vi "Keithley 2600 Series Read Resistance Measurement.vi"() -> ()   [LabVIEW 2020]
doc: "This example shows how to configure the source output, source measurement and perform one resistance measurement."
uses:
  <instrlib>/Keithley 2600 Series/Public/Configure/Source/Configure Source (Range).vi
  <instrlib>/Keithley 2600 Series/Public/Configure/Source/Configure Source (Level).vi
  <instrlib>/Keithley 2600 Series/Public/Configure/Source/Configure Source (Limit).vi
  <instrlib>/Keithley 2600 Series/Public/Data/Read Measurement (Resistance).vi
  <instrlib>/Keithley 2600 Series/Keithley 2600 Series.lvlib
panel:
  out "Resistance (Ohm)":dbl
  in  "Sense Mode (0: Local Sense)":i32(ring) items=["Local Sense", "Remote Sense"]
  in  "Voltage Limit (5 V)":dbl=5.0
  in  "Current Level (0.1 A)":dbl=0.1
  in  "Current Range (0.1 A)":dbl=0.1
  in  "Source Function (0: Current)":i32(ring) items=["Current"]
  in  "Source Measure Unit Channel (0: Channel A)":i32(ring) items=["Channel A", "Channel B"]
  in  "VISA resource name":refnum<visa-resource-name>
  # "(c) 2020 National Instruments.  ALL RIGHTS RESERVED."
  # "Measurement Result"
  # "Source Output Configuration"
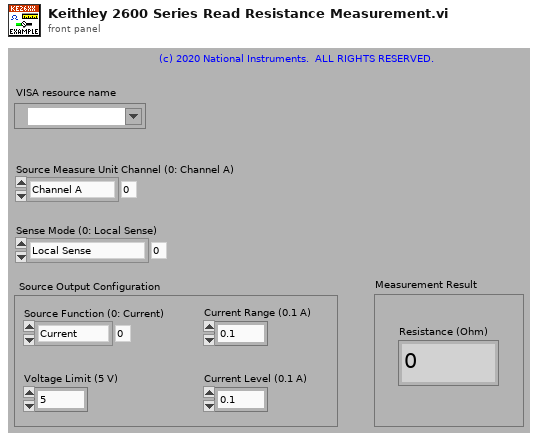
[diagram p1: front panel]
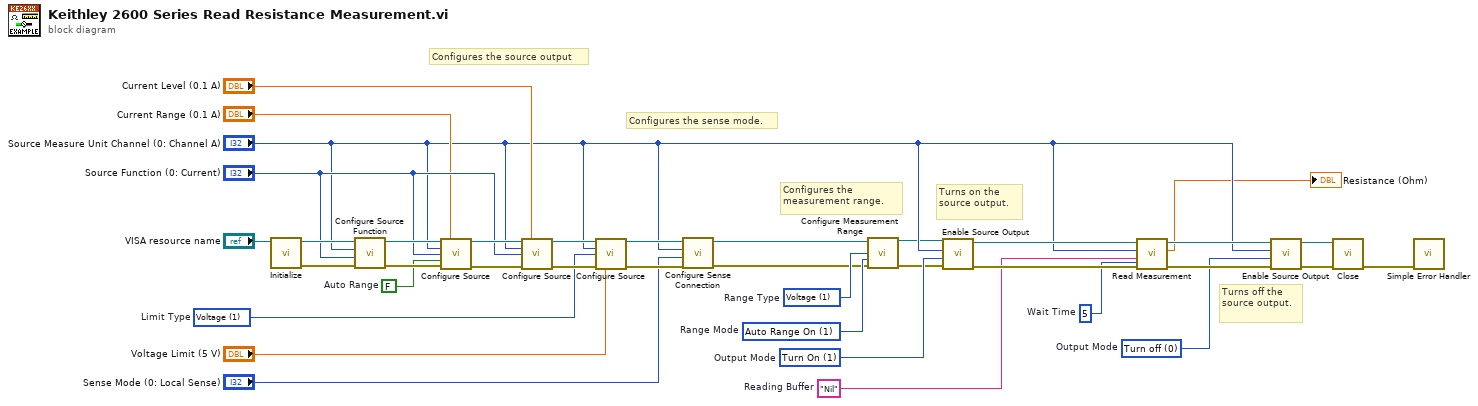
[diagram p0: block diagram]
diagram:
  w1 = 1 items=["Current", "Voltage", "Power"]  # Limit Type
  w9 = 1 items=["Auto Range Off", "Auto Range On", "Auto Range Follow Limit"]  # Range Mode
  w10 = 1 items=["Current", "Voltage"]  # Range Type
  w19 = 0 items=["Turn off", "Turn On", "High-Z"]  # Output Mode
  w22 = 5  # Wait Time
  w26 = 1 items=["Turn off", "Turn On", "High-Z"]  # Output Mode
  w23 = "Nil"  # Reading Buffer
  w30 = FALSE  # Auto Range
  # "Configures the measurement range."
  # "Configures the sense mode."
  # "Turns off the source output."
  # "Turns on the source output."
  # "Configures the source output"
  n1 = call <instrlib>:"Initialize.vi"("VISA resource name"="VISA resource name") -> ("error out"=w35:errorcluster, "VISA resource name out"=w36:refnum<visa-resource-name>)  [unwired: 9 in]
  n2 = call <instrlib>:"Configure Source Function.vi"("error in (no error)"=w35, "Source Function (1: Voltage)"="Source Function (0: Current)", "Source Measure Unit Channel (0: Channel A)"="Source Measure Unit Channel (0: Channel A)", "VISA resource name"=w36) -> ("error out"=w33:errorcluster, "VISA resource name out"=w34:refnum<visa-resource-name>)  [unwired: 6 in]
  n3 = call-poly <instrlib>:"Configure Source.vi"("VISA resource name"=w34, "Current Range (1E-7 A)"="Current Range (0.1 A)", "Source Measure Unit Channel (0: Channel A)"="Source Measure Unit Channel (0: Channel A)", "Range Type (1: Voltage)"="Source Function (0: Current)", "Auto Range (T: Enable)"=w30, "error in (no error)"=w33) -> ("VISA resource name out"=w32:refnum<visa-resource-name>, "error out"=w31:errorcluster)  [unwired: 8 in]
  n4 = call-poly <instrlib>:"Configure Source.vi"("VISA resource name"=w32, "Current Level (0 A)"="Current Level (0.1 A)", "Source Measure Unit Channel (0: Channel A)"="Source Measure Unit Channel (0: Channel A)", "Level Type (1: Voltage)"="Source Function (0: Current)", "error in (no error)"=w31) -> ("VISA resource name out"=w29:refnum<visa-resource-name>, "error out"=w28:errorcluster)  [unwired: 9 in]
  n5 = call-poly <instrlib>:"Configure Source.vi"("VISA resource name"=w29, "Source Measure Unit Channel (0: Channel A)"="Source Measure Unit Channel (0: Channel A)", "Limit Type (1: Voltage)"=w1, "error in (no error)"=w28, "Voltage Limit (20 V)"="Voltage Limit (5 V)") -> ("VISA resource name out"=w15:refnum<visa-resource-name>, "error out"=w14:errorcluster)  [unwired: 9 in]
  n6 = call <instrlib>:"Configure Sense Connection.vi"("error in (no error)"=w14, "Sense Mode (0: Local Sense)"="Sense Mode (0: Local Sense)", "Source Measure Unit Channel (0: Channel A)"="Source Measure Unit Channel (0: Channel A)", "VISA resource name"=w15) -> ("error out"=w5:errorcluster, "VISA resource name out"=w6:refnum<visa-resource-name>)  [unwired: 6 in]
  n7 = call <instrlib>:"Configure Measurement Range.vi"("VISA resource name"=w6, "Range Type (0: Current)"=w10, "Range Mode (1: Auto Range On)"=w9, "error in (no error)"=w5) -> ("VISA resource name out"=w8:refnum<visa-resource-name>, "error out"=w7:errorcluster)  [unwired: 10 in]
  n8 = call <instrlib>:"Enable Source Output.vi"("error in (no error)"=w7, "Output Mode (0: Turn off)"=w26, "Source Measure Unit Channel (0: Channel A)"="Source Measure Unit Channel (0: Channel A)", "VISA resource name"=w8) -> ("error out"=w24:errorcluster, "VISA resource name out"=w25:refnum<visa-resource-name>)  [unwired: 6 in]
  n9 = call-poly <instrlib>:"Read Measurement.vi"("Wait Time (10 S)"=w22, "error in (no error)"=w24, "Resistance Buffer (smua.nvbuffer1)"=w23, "Source Measure Unit Channel (0: Channel A)"="Source Measure Unit Channel (0: Channel A)", "VISA resource name"=w25) -> ("error out"=w20:errorcluster, "Last Resistance (Ohm)"=→"Resistance (Ohm)":dbl, "VISA resource name out"=w21:refnum<visa-resource-name>)  [unwired: 3 in, 1 out]
  n10 = call <instrlib>:"Enable Source Output.vi"("error in (no error)"=w20, "Output Mode (0: Turn off)"=w19, "Source Measure Unit Channel (0: Channel A)"="Source Measure Unit Channel (0: Channel A)", "VISA resource name"=w21) -> ("error out"=w3:errorcluster, "VISA resource name out"=w4:refnum<visa-resource-name>)  [unwired: 6 in]
  n11 = call <instrlib>:"Close.vi"("error in (no error)"=w3, "VISA resource name"=w4) -> ("error out"=w2:errorcluster)  [unwired: 9 in]
  n12 = call <vilib>:"Simple Error Handler.vi"("error in (no error)"=w2) -> ()  [unwired: 4 in, 5 out]
